vi "deviation region.vi"(9 "dev margin":dbl=1.0, 10 "dev bounds":T1, 11 "dev point":T2={"dev point cap (100)"=100.0, "dev point loss (0)"=0.0}) -> (2 "deviation region":cluster{cluster{dbl, dbl}[]}[](graph))   [LabVIEW 2019, in "Andeen-Hagerling 2700A.lvlib"]
doc: "Generate a graph representing the deviation region."
uses:
  Andeen-Hagerling 2700A.lvlib
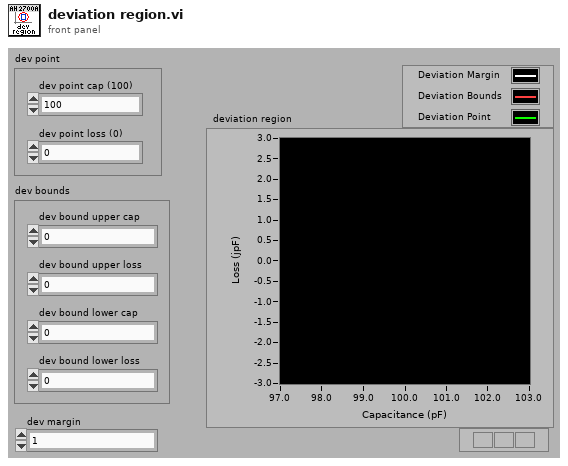
[diagram p1: front panel]
types:
  T1 = cluster{"dev bound upper cap":dbl, "dev bound upper loss":dbl, "dev bound lower cap":dbl, "dev bound lower loss":dbl}
  T2 = cluster{"dev point cap (100)":dbl, "dev point loss (0)":dbl}
  T3 = cluster{cluster{"dev point cap (100)":dbl, "dev point loss (0)":dbl}[]}
  T4 = cluster{cluster{"dev point cap (100)":dbl, "dev point loss (0)":dbl}[]}[]
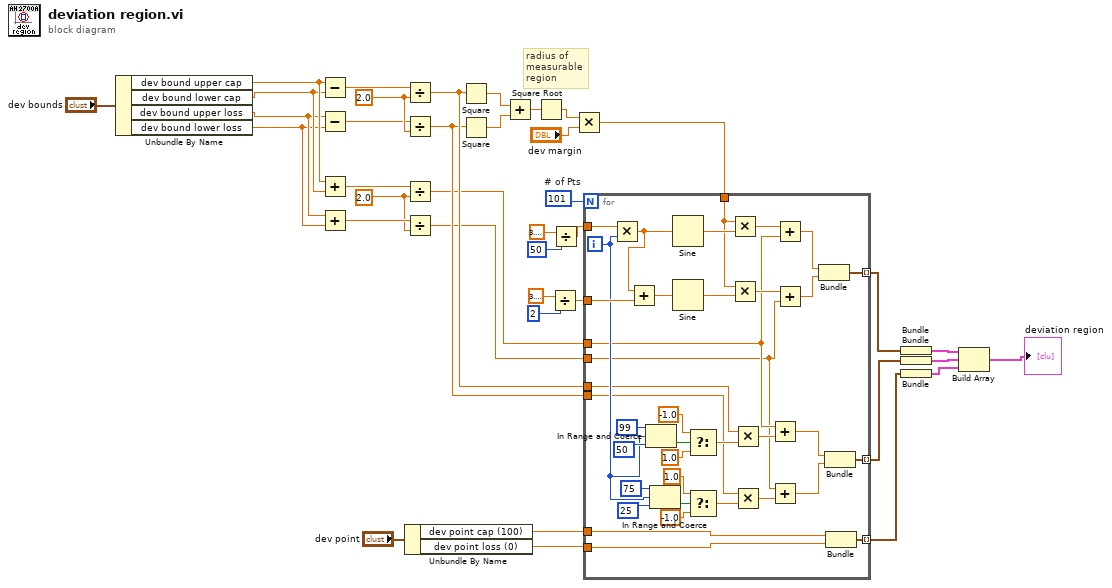
[diagram p0: block diagram]
diagram:
  w9 = 2.0 ("y")
  w25 = 2.0 ("y")
  w38 = 101  # # of Pts
  # "radius of\nmeasurable\nregion"
  n1 = Unbundle By Name("dev bounds") -> ("dev bound upper cap"=w8:dbl, "dev bound lower cap"=w7:dbl, "dev bound upper loss"=w6:dbl, "dev bound lower loss"=w5:dbl)
  n2 = Subtract(x=w8, y=w7) -> (x-y=w13:dbl)
  n3 = Subtract(x=w6, y=w5) -> (x-y=w12:dbl)
  n4 = Add(x=w8, y=w7) -> (x+y=w10:dbl)
  n5 = Add(x=w6, y=w5) -> (x+y=w11:dbl)
  n6 = Divide(x=w13, y=w25) -> (x/y=w21:dbl)
  n7 = Divide(x=w12, y=w25) -> (x/y=w20:dbl)
  n8 = Divide(x=w10, y=w9) -> (x/y=w4:dbl)
  n9 = Divide(x=w11, y=w9) -> (x/y=w3:dbl)
  n10 = Unbundle By Name("dev point") -> ("dev point cap (100)"=w2:dbl, "dev point loss (0)"=w1:dbl)
  n11 = Square(x=w21) -> (x^2=w30:dbl)
  n12 = Square(x=w20) -> (x^2=w31:dbl)
  n13 = Add(x=w30, y=w31) -> (x+y=w29:dbl)
  n14 = Square Root(x=w29) -> (sqrt(x)=w27:dbl)
  n15 = Divide(x=3.141592653589793, y=2) -> (x/y=w32:dbl)
  n16 = Divide(x=3.141592653589793, y=50) -> (x/y=w36:dbl)
  n17 = Multiply(x=w27, y="dev margin") -> (x*y=w26:dbl)
  n18 = for {
    N: w38 -> [_]
    tunnel: w36 -> [w75]
    tunnel: [w74] -> w19 mode=indexing
    tunnel: w32 -> [w73]
    tunnel: w26 -> [w68]
    tunnel: w4 -> [w42]
    tunnel: w3 -> [w41]
    tunnel: w21 -> [w45]
    tunnel: w20 -> [w44]
    tunnel: [w46] -> w18 mode=indexing
    tunnel: [w43] -> w15 mode=indexing
    tunnel: w2 -> [w40]
    tunnel: w1 -> [w39]
    i -> [w53]
    n19 = Multiply(x=w75, y=w53) -> (x*y=w72:dbl)
    n20 = Add(x=w72, y=w73) -> (x+y=w71:dbl)
    n21 = In Range and Coerce(upper limit=99, x=w53, lower limit=50) -> (In Range?=w61:bool)  [unwired: 1 out]
    n22 = In Range and Coerce(upper limit=75, x=w53, lower limit=25) -> (In Range?=w56:bool)  [unwired: 1 out]
    n23 = Sine(x=w72) -> (sin(x)=w70:dbl)
    n24 = Sine(x=w71) -> (sin(x)=w69:dbl)
    n25 = Select(t=-1.0, s=w61, f=1.0) -> (s? t:f=w52:dbl)
    n26 = Select(t=1.0, s=w56, f=-1.0) -> (s? t:f=w50:dbl)
    n27 = Multiply(x=w68, y=w70) -> (x*y=w67:dbl)
    n28 = Multiply(x=w68, y=w69) -> (x*y=w66:dbl)
    n29 = Multiply(x=w45, y=w52) -> (x*y=w51:dbl)
    n30 = Multiply(x=w44, y=w50) -> (x*y=w49:dbl)
    n31 = Add(x=w42, y=w51) -> (x+y=w48:dbl)
    n32 = Add(x=w41, y=w49) -> (x+y=w47:dbl)
    n33 = Add(x=w67, y=w42) -> (x+y=w65:dbl)
    n34 = Add(x=w66, y=w41) -> (x+y=w64:dbl)
    n35 = Bundle "Bundle"(w65, w64) -> (w74:cluster{dbl, dbl})  [unwired: 1 in]
    n36 = Bundle "Bundle"(w48, w47) -> (w46:cluster{dbl, dbl})  [unwired: 1 in]
    n37 = Bundle "Bundle"("dev point cap (100)"=w40, "dev point loss (0)"=w39) -> (w43:T2)  [unwired: 1 in]
  }
  n38 = Bundle "Bundle"(w19) -> (w24:cluster{cluster{dbl, dbl}[]})  [unwired: 1 in]
  n39 = Bundle(w18) -> (w23:cluster{cluster{dbl, dbl}[]})  [unwired: 1 in]
  n40 = Bundle(w15) -> (w16:T3)  [unwired: 1 in]
  n41 = Build Array "Build Array"(w24, w23, w16) -> (→"deviation region":T4)
